vi "Configure and Start Housekeeping.vi"(8 "error in":errorcluster, 11 "cPAS in":refnum<class "cPAS.lvclass">) -> (0 "error out":errorcluster, 3 "cPAS out":refnum<class "cPAS.lvclass">)   [LabVIEW 2015, in "cPAS.lvclass"]
uses:
  cPAS.lvclass
  cPAS.lvclass/cPAS.ctl
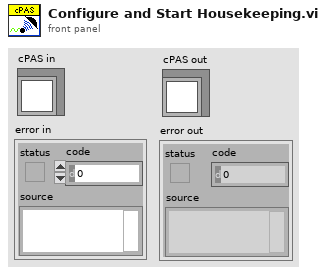
[diagram p1: front panel]
types:
  T1 = cluster{"Cell 1":bool, "Cell 2":bool, "Cell 3":bool, "Cell 4":bool, "Cell 5":bool}
  T2 = cluster{"Cell 1":sgl, "Cell 2":sgl, "Cell 3":sgl, "Cell 4":sgl, "Cell 5":sgl}
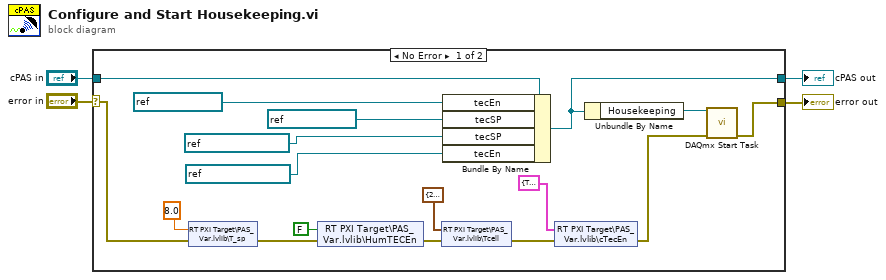
[diagram p0: block diagram]
diagram:
  n1 = case shown="No Error" "error in" {
    selector: "error in" -> [w9 w22]
    tunnel: [w6 w22] -> w4
    tunnel: [w7 w23] -> w3
    tunnel: "cPAS in" -> [w20 w23]
    frame No Error {
      n2 = shared-variable "RT PXI Target\\PAS_Var.lvlib\\T_sp"(sgl 8.0 ("T_sp"), error in=w9) -> (error out=w14:errorcluster)
      n3 = shared-variable "RT PXI Target\\PAS_Var.lvlib\\HumTECEn"(FALSE ("HumTECEn"), error in=w14) -> (error out=w10:errorcluster)
      n4 = shared-variable "RT PXI Target\\PAS_Var.lvlib\\Tcell"(T2 {"Cell 1"=21.0, "Cell 2"=21.0, "Cell 3"=21.0, "Cell 4"=21.0, "Cell 5"=24.0} ("Tcell"), error in=w10) -> (error out=w21:errorcluster)
      n5 = Bundle By Name(cluster=w20, "tecEn"=refnum<k21> "PAS TEC En", "tecSP"=refnum<k21> "PAS TEC SP", "tecSP"=refnum<k21> "PAS Hum T SP", "tecEn"=refnum<k21> "PAS Hum T En" ("tecSP")) -> (w7:refnum<class "cPAS.lvclass">)
      n6 = shared-variable "RT PXI Target\\PAS_Var.lvlib\\cTecEn"(T1 {"Cell 1"=TRUE, "Cell 2"=TRUE, "Cell 3"=TRUE, "Cell 4"=TRUE, "Cell 5"=TRUE} ("cTecEn"), error in=w21) -> (error out=w5:errorcluster)
      n7 = Unbundle By Name(w7) -> ("Housekeeping"=w8:refnum<k21>)
      n8 = call <vilib>:"DAQmx Start Task.vi"("task/channels in"=w8, "error in"=w5) -> ("error out"=w6:errorcluster)  [unwired: 12 in, 1 out]
    }
    frame Error {
    }
  }
  "error out" <- w4
  "cPAS out" <- w3
